vi "Write Exp selector ref.vi"(8 "error in (no error)":errorcluster, 10 "Exp selector ref":refnum<vi>, 11 "Control-Client in":refnum<class "Control-Client.lvclass">) -> (0 "error out":errorcluster, 3 "Control-Client out":refnum<class "Control-Client.lvclass">)   [LabVIEW 2019, in "Control-Client.lvclass"]
uses:
  Control-Client.lvclass
  controls/mylistbox.ctl
  Control-Client.lvclass/Control-Client.ctl
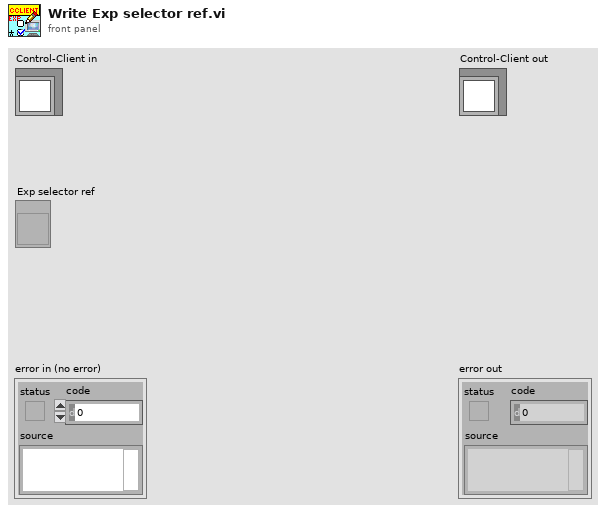
[diagram p1: front panel]
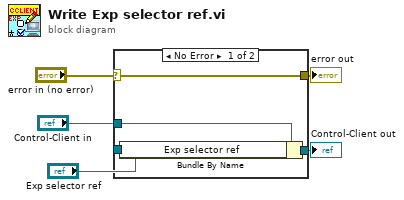
[diagram p0: block diagram]
diagram:
  n1 = case shown="No Error" "error in (no error)" {
    selector: "error in (no error)" -> [w9 w10]
    tunnel: [w9 w10] -> w4
    tunnel: [w7 w11] -> w2
    tunnel: "Control-Client in" -> [w8 w11]
    tunnel: "Exp selector ref" -> [w6 _]
    frame No Error {
      n2 = Bundle By Name(cluster=w8, "Exp selector ref"=w6) -> (w7:refnum<class "Control-Client.lvclass">)
    }
    frame Error {
    }
  }
  "error out" <- w4
  "Control-Client out" <- w2
